vi "DELETE Request.vi"(8 "error in (no error)":errorcluster, 10 "Path (after URL)":string, 11 "REST Interface in":refnum<class "REST Interface.lvclass">) -> (0 "error out":errorcluster, 1 "Status Code":u16, 2 "Response":string, 3 "REST Interface out":refnum<class "REST Interface.lvclass">)   [LabVIEW 2018, in "REST Interface.lvlib" / "REST Interface.lvclass"]
uses:
  REST Interface.lvclass
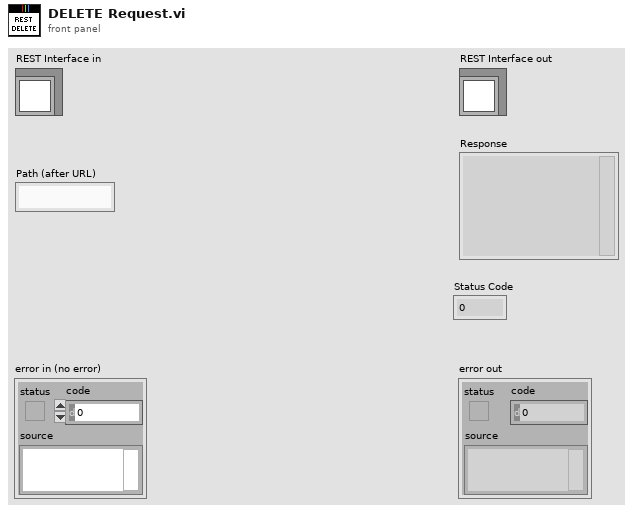
[diagram p1: front panel]
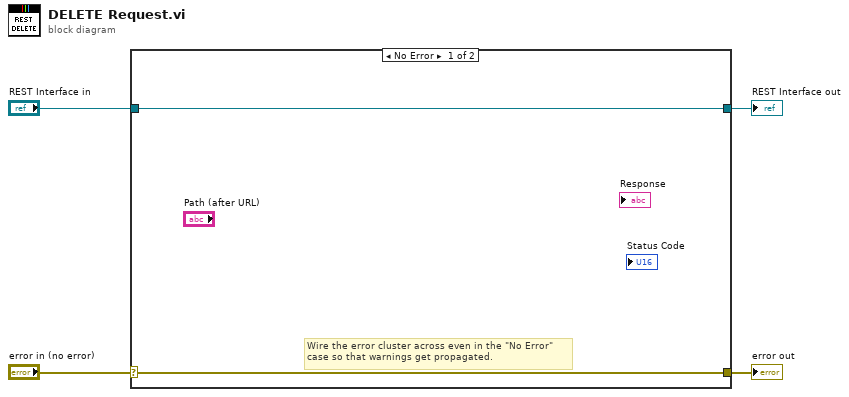
[diagram p0: block diagram]
diagram:
  n1 = case shown="No Error" "error in (no error)" {
    selector: "error in (no error)" -> [w5 w8]
    tunnel: [w5 w8] -> w3
    tunnel: [w6 w7] -> w1
    tunnel: "REST Interface in" -> [w6 w7]
    frame No Error {
      # "Wire the error cluster across even in the \"No Error\"\ncase so that warnings get propagated."
    }
    frame Error {
    }
  }
  "error out" <- w3
  "REST Interface out" <- w1
